vi "Request Background Movement Correction STOP.vi"(8 "error in (no error)":errorcluster, 9 "Next State":T1, 11 "UI queue in":refnum<queue>) -> (0 "error out":errorcluster, 3 "UI queue out":refnum<queue>)   [LabVIEW 2020]
uses:
  Queue/Message Queue/Typedefs/Message Cluster.ctl
  Typedefs/Top level VI states.ctl
  Typedefs/Start-Stop Enum.ctl
panel:
  in  "milliseconds to wait":u32=10
  # "<---See description"
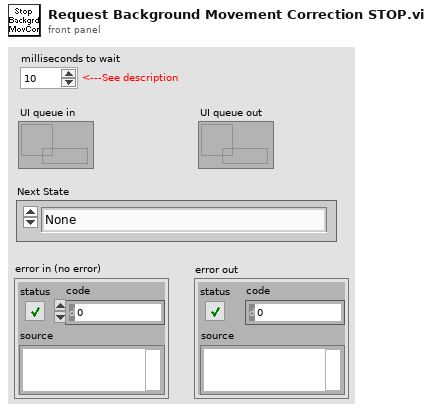
[diagram p1: front panel]
types:
  T1 = typedef "Top level VI states.ctl" = enum16{"None", "Initialise UI", "<STACK PROTOCOL STATES>", "AOL Zstack-START", "AOL Zstack-STOP", "Motor Zstack-START", "Motor Zstack-STOP", "<ACQUISITION PROTOCOL STATES> ", "Functional Acquisition-START", "Functional Acquisition-STOP", "Single Plane Acquisition-START", "Single Plane Acquisition-STOP", "Volume Acquisition-START", "Volume Acquisition-STOP", "<LIVE IMAGING PROTOCOL STATES>", "Live Imaging-START", "Live Imaging-STOP", "Live Plane Imaging-START", "Live Plane Imaging-STOP", "Live Volume Imaging-START", "Live Volume Imaging-STOP", "<MOVEMENT CORRECTION PROTOCOL STATES>", "EXIT"}
  T2 = typedef "Start-Stop Enum.ctl" = enum16{"START", "STOP"}
  T3 = typedef "Top level VI states.ctl" = enum16{"None", "Initialise UI", "<STACK PROTOCOL STATES>", "AOL Zstack-START", "AOL Zstack-STOP", "Motor Zstack-START", "Motor Zstack-STOP", "<ACQUISITION PROTOCOL STATES> ", "Functional Acquisition-START", "Functional Acquisition-STOP", "Single Plane Acquisition-START", "Single Plane Acquisition-STOP", "Volume Acquisition-START", "Volume Acquisition-STOP", "<LIVE IMAGING PROTOCOL STATES>", "Live Imaging-START", "Live Imaging-STOP", "Live Plane Imaging-START", "Live Plane Imaging-STOP", "Live Volume Imaging-START", "Live Volume Imaging-STOP", "<MOVEMENT CORRECTION PROTOCOL STATES>", "Background MovCor-START", "Background MovCor-STOP", "EXIT"}
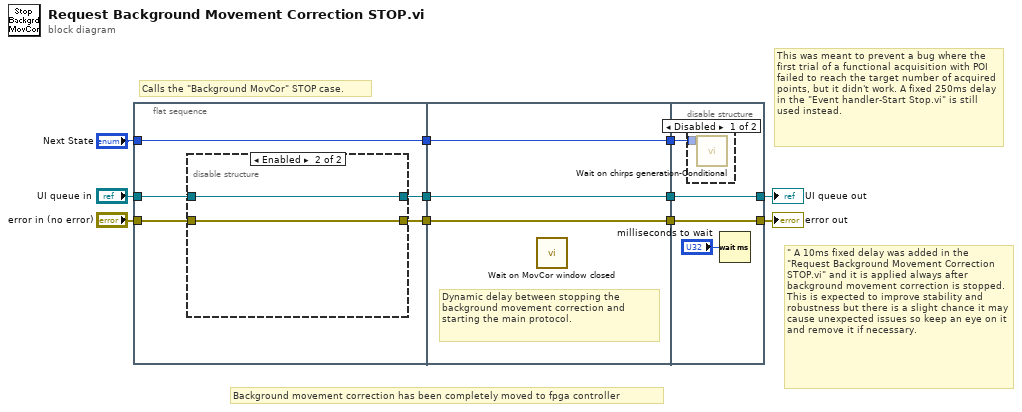
[diagram p0: block diagram]
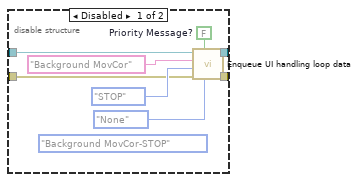
[diagram p2: hidden frame]
diagram:
  # "Background movement correction has been completely moved to fpga controller"
  # "\"\tA 10ms fixed delay was added in the \"Request Background Movement Correction STOP.vi\" and it is applied always after background movement correction is stopped. This is expected to improve stability and robustness but there is a slight chance it may cause unexpected issues so keep an eye on it and remove it if necessary."
  # "This was meant to prevent a bug where the first trial of a functional acquisition with POI failed to reach the target number of acquired points, but it didn't work. A fixed 250ms delay in the \"Event handler-Start Stop.vi\" is still used instead."
  # "Calls the \"Background MovCor\" STOP case."
  n1 = flat-sequence {
    tunnel: "UI queue in" -> [w16]
    tunnel: "error in (no error)" -> [w13]
    tunnel: [w15] -> w7
    tunnel: [w14] -> w6
    tunnel: "Next State" -> [w12]
    tunnel: [w12] -> w4
    tunnel: w7 -> [w29]
    tunnel: w6 -> [w28]
    tunnel: w4 -> [w27]
    tunnel: [w29] -> w3
    tunnel: [w28] -> w2
    tunnel: [w27] -> w1
    tunnel: [w32] -> w9
    tunnel: [w33] -> w10
    tunnel: w3 -> [w33]
    tunnel: w2 -> [w32]
    tunnel: w1 -> [w31]
    frame #0 {
      n2 = disable-structure shown="Enabled" {
        disable-tunnel: w16 -> [w23 w26]
        disable-tunnel: [w21 w26] -> w15
        disable-tunnel: [w20 w25] -> w14
        disable-tunnel: w13 -> [w19 w25]
        frame Disabled {
          w18 = FALSE  # Priority Message?
          (unwired) Top_level_VI_states."Background MovCor-STOP" ("Next State")
          n3 = call "Enqueue UI handling loop data.vi"("Next State"=Top_level_VI_states."None", "Priority Message? (T)"=w18, "error in (no error)"=w19, "Start/Stop"=Start-Stop_Enum."STOP", "Message"="Background MovCor", "Queue in"=w23) -> ("error out"=w20:errorcluster, "Queue out"=w21:refnum<queue>)  [unwired: 4 in]
        }
        frame Enabled {
        }
      }
    }
    frame #1 {
      # "Dynamic delay between stopping the background movement correction and starting the main protocol."
      n4 = call "Wait on MovCor window closed.vi"() -> ()  [unwired: 11 in, 1 out]
    }
    frame #2 {
      n5 = disable-structure shown="Disabled" {
        disable-tunnel: w31 -> [w34 _]
        frame Disabled {
          n6 = call "Wait on chirps generation-Conditional.vi"("Next State"=w34) -> ()  [unwired: 9 in, 2 out]
        }
        frame Enabled {
        }
      }
      n7 = Wait (ms)(milliseconds to wait="milliseconds to wait") -> ()  [unwired: 1 out]
    }
  }
  "UI queue out" <- w10
  "error out" <- w9
